vi "hwOperation_ReadData.vi"(6 "t0":timestamp, 7 "hwType":string, 8 "error in":errorcluster, 10 "Devs Info in":T1[](array[typedef]), 11 "hwDriverRef in":T3) -> (0 "error out":errorcluster, 1 "Waveform[]":waveform(dbl)[](array[waveform]), 3 "hwDriverRef out":T3, 4 "t0":timestamp)   [LabVIEW 2016]
uses:
  QX/hw_QX_hwDriverRef.ctl
  C:/Users/CL/Desktop/ZcDAQprj0811/ZcDAQprj/Modules/DAQ-Device/Hardware Drivers/QX/HBM LabVIEW Driver/DLLs/Hbm.Api.Common.dll
  QX/HBM LabVIEW Driver/DLLs/Hbm.Api.Common.dll
  DAQ-Config/Controls/PSCHN_Card Para.ctl
  DAQ-Config/Controls/PSCHN_Channel Para.ctl
  <vilib>/measure/NI_MABase.lvlib
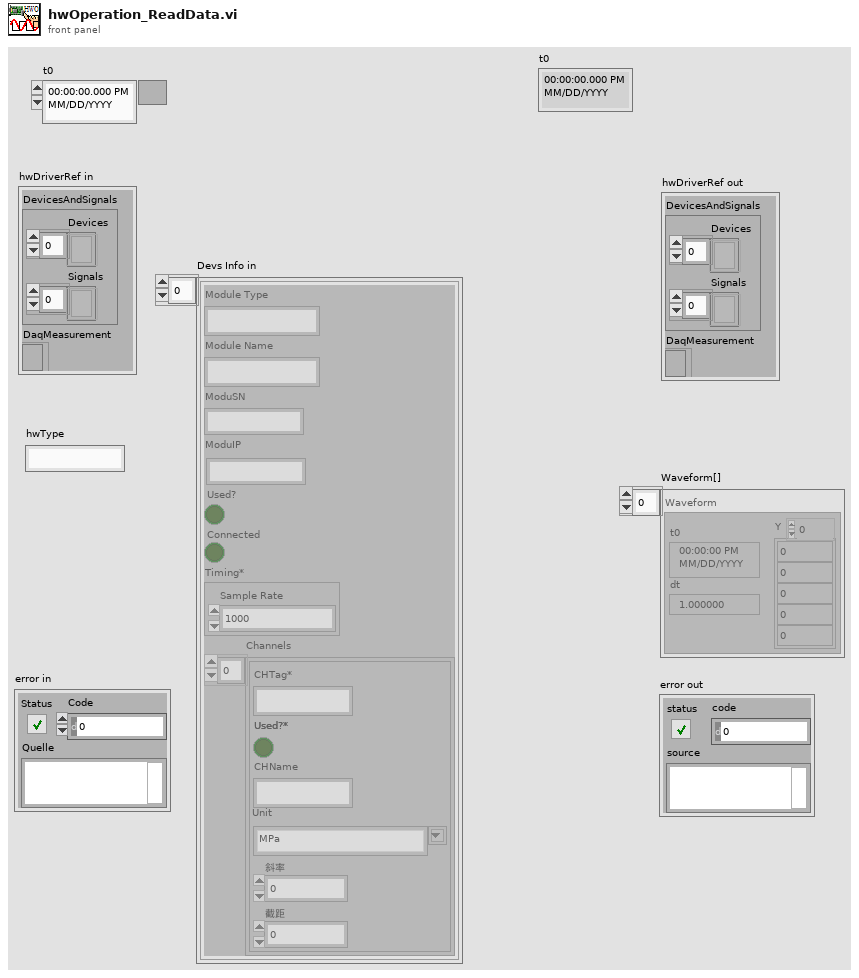
[diagram p1: front panel]
types:
  T1 = typedef "PSCHN_Card Para.ctl" = cluster{"Module Type":string, "Module Name":string, "ModuSN":string, "ModuIP":string, "Used?":bool, "Connected":bool, "Timing*":cluster{"Sample Rate":dbl}, "Channels":T2[]}
  T2 = typedef "PSCHN_Channel Para.ctl" = cluster{"CHTag*":string, "Used?*":bool, "CHName":string, "Unit":string, "斜率":dbl, "截距":dbl}
  T3 = typedef "hw_QX_hwDriverRef.ctl" = cluster{"DevicesAndSignals":cluster{"Devices":refnum<k24>[], "Signals":refnum<k24>[]}, "DaqMeasurement":refnum<k24>}
  T4 = enum16{"Sine Wave", "Triangle Wave", "Square Wave", "Sawtooth Wave"}
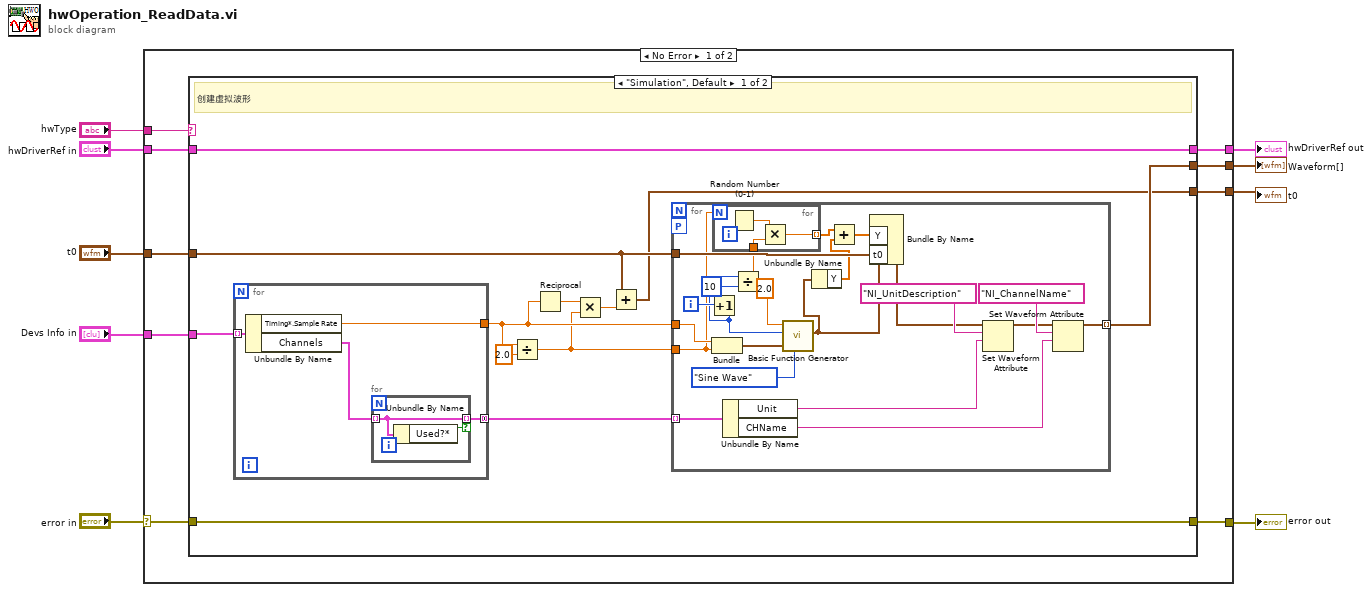
[diagram p0: block diagram]
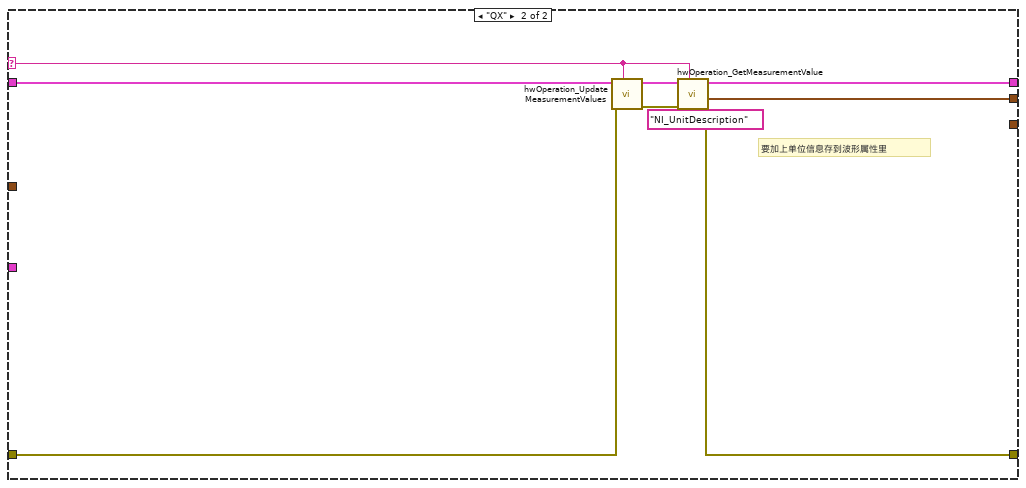
[diagram p2: hidden frame]
diagram:
  n1 = case shown="No Error" "error in" {
    selector: "error in" -> [w17 w71]
    tunnel: [w18 w71] -> w8
    tunnel: "hwType" -> [w16 _]
    tunnel: "hwDriverRef in" -> [w15 w70]
    tunnel: [w14 w70] -> w5
    tunnel: [w13 _] -> w4
    tunnel: "Devs Info in" -> [w12 _]
    tunnel: "t0" -> [w11 _]
    tunnel: [w10 _] -> w1
    frame No Error {
      n2 = case shown="\"Simulation\", Default" w16 {
        selector: w16 -> [_ w66]
        tunnel: [w30 w68] -> w18
        tunnel: w17 -> [w30 w65]
        tunnel: w15 -> [w29 w64]
        tunnel: [w29 w63] -> w14
        tunnel: [w28 w62] -> w13
        tunnel: w12 -> [w27 _]
        tunnel: w11 -> [w20 _]
        tunnel: [w19 _] -> w10
        frame "Simulation", Default {
          # "创建虚拟波形"
          n3 = for {
            tunnel: w27 -> [w59] mode=indexing
            tunnel: [w56] -> w26 mode=concatenating
            tunnel: [w58] -> w24
            n4 = Unbundle By Name(w59) -> ("Timing*.Sample Rate"=w58:dbl, "Channels"=w57:T2[])
            n5 = for {
              tunnel: w57 -> [w61] mode=indexing
              tunnel: [w61] -> w56 mode=indexing if=w60
              n6 = Unbundle By Name(w61) -> ("Used?*"=w60:bool)
            }
          }
          n7 = Divide(x=w24, y=2.0) -> (x/y=w22:dbl)
          n8 = Reciprocal(x=w24) -> (1/x=w23:dbl)
          n9 = Multiply(x=w23, y=w22) -> (x*y=w21:dbl)
          n10 = Add(x=w20, y=w21) -> (x+y=w19:timestamp)
          n11 = for {
            tunnel: w24 -> [w51]
            tunnel: w22 -> [w39]
            tunnel: w26 -> [w48] mode=indexing
            tunnel: [w46] -> w28 mode=indexing
            workers-P: _ -> [_]
            tunnel: w20 -> [w40]
            i -> [w45]
            n12 = Increment(x=w45) -> (x+1=w37:i32)
            n13 = Bundle("Sample Rate"=w51, w39) -> (w49:cluster{"Sample Rate":dbl, dbl})  [unwired: 1 in]
            n14 = Unbundle By Name(w48) -> ("Unit"=w43:string, "CHName"=w47:string)
            n15 = Divide(x=w37, y=10) -> (x/y=w35:dbl)
            n16 = for {
              N: w39 -> [_]
              tunnel: [w54] -> w32 mode=indexing
              tunnel: w35 -> [w53]
              n17 = Random Number (0-1)() -> (number: 0 to 1=w55:dbl)
              n18 = Multiply(x=w55, y=w53) -> (x*y=w54:dbl)
            }
            n19 = call <vilib>:"Basic Function Generator.vi"("sampling info"=w49, "signal type"=T4."Sine Wave", "amplitude"=w37, "frequency"=2.0) -> ("signal out"=w34:waveform(dbl))  [unwired: 5 in, 2 out]
            n20 = Unbundle By Name(w34) -> ("Y"=w33:dbl[])
            n21 = Add(x=w32, y=w33) -> (x+y=w31:dbl[])
            n22 = Bundle By Name(cluster=w34, "Y"=w31, "t0"=w40) -> (w41:waveform(dbl))
            n23 = Set Waveform Attribute(5:w43, 6:"NI_UnitDescription" ("名称"), 7:w41) -> (3:w44:waveform(dbl))  [unwired: 1 in, 2 out]
            n24 = Set Waveform Attribute(5:w47, 6:"NI_ChannelName" ("Channel Name"), 7:w44) -> (3:w46:waveform(dbl))  [unwired: 1 in, 2 out]
          }
        }
        frame "QX" {
          (unwired) "NI_UnitDescription" ("名称")
          # "要加上单位信息存到波形属性里"
          n25 = call "hwOperation_Update MeasurementValues.vi"("hwType"=w66, "Error in"=w65, "hwDriverRef in"=w64) -> ("Error out"=w69:errorcluster, "hwDriverRef out"=w67:T3)  [unwired: 7 in]
          n26 = call "hwOperation_GetMeasurementValue.vi"("hwType"=w66, "Error in"=w69, "hwDriverRef in"=w67) -> ("Error out"=w68:errorcluster, "Waveform[]"=w62:waveform(dbl)[], "hwDriverRef out"=w63:T3)  [unwired: 3 in, 3 out]
        }
      }
    }
    frame Error {
    }
  }
  "error out" <- w8
  "hwDriverRef out" <- w5
  "Waveform[]" <- w4
  "t0" <- w1
